vi "Read right SR.vi"(9 "ShiftRegister in":refnum<class "ShiftRegister.lvclass">) -> (3 "ShiftRegister out":refnum<class "ShiftRegister.lvclass">, 4 "right SR":refnum<class "RightShiftRegister.lvclass">)   [LabVIEW 2014, in "ShiftRegister.lvclass"]
uses:
  ShiftRegister.lvclass
  RightShiftRegister/RightShiftRegister.lvclass
  ShiftRegister.lvclass/ShiftRegister.ctl
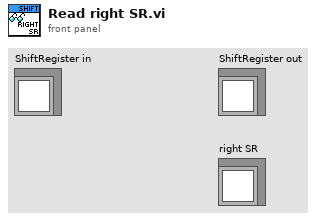
[diagram p1: front panel]
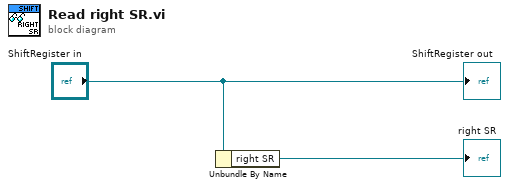
[diagram p0: block diagram]
diagram:
  n1 = Unbundle By Name("ShiftRegister in") -> ("right SR"=→"right SR":refnum<class "RightShiftRegister.lvclass">)
  "ShiftRegister out" <- "ShiftRegister in"
